vi "Delete QDFunction.vi"(8 "error in (no error)":errorcluster, 10 "QDFullName(\"\")":string, 11 "ScriptSetting in":refnum<class "ScriptSetting.lvclass">) -> (0 "error out":errorcluster, 3 "ScriptSetting out":refnum<class "ScriptSetting.lvclass">)   [LabVIEW 2015, in "ScriptSetting.lvclass"]
uses:
  ScriptSetting.lvclass
  ScriptSetting.lvclass/ScriptSetting.ctl
  QDSearchList/QDDialogList.lvclass/QDDialogList.ctl
  _Database/Implements/ScriptDatabase.lvclass/ScriptDatabase.ctl
  <vilib>/Utility/error.llb/Error Cluster From Error Code.vi
  <vilib>/ErrorRing/Error Ring.xnode
  QDSearchList/QDDialogList.lvclass
  _Database/Implements/ScriptDatabase.lvclass
  _Database/Ancestor/DatabaseAPI.lvclass
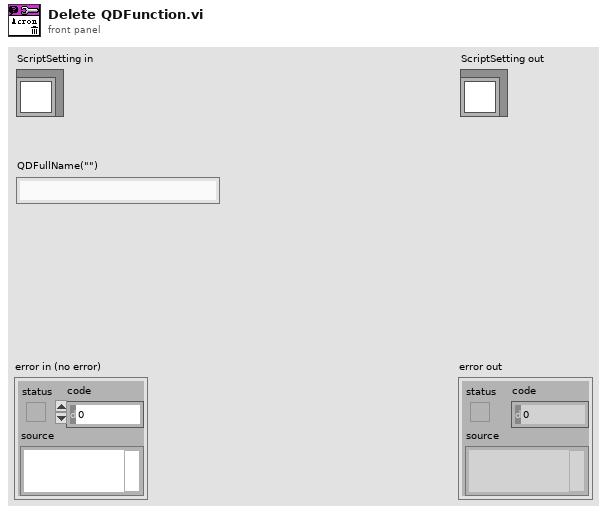
[diagram p1: front panel]
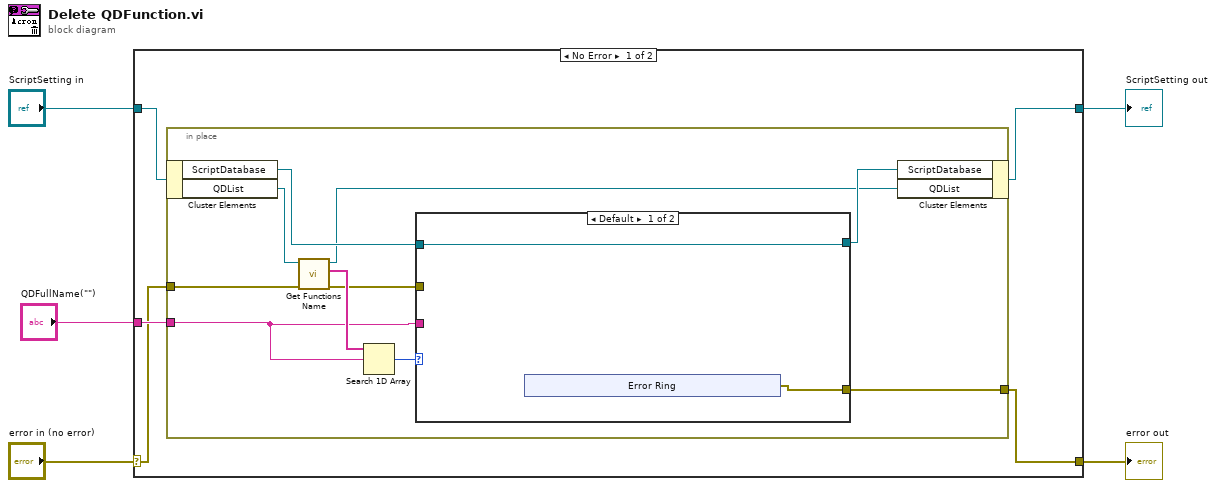
[diagram p0: block diagram]
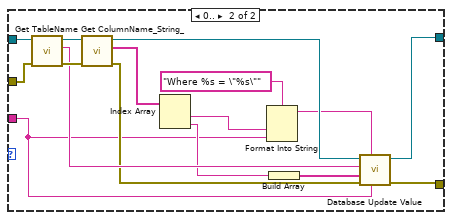
[diagram p2: hidden frame]
diagram:
  n1 = case shown="No Error" "error in (no error)" {
    selector: "error in (no error)" -> [w8 w45]
    tunnel: [w7 w45] -> w4
    tunnel: [w6 w44] -> w2
    tunnel: "ScriptSetting in" -> [w10 w44]
    tunnel: "QDFullName(\"\")" -> [w9 _]
    frame No Error {
      n2 = in-place {
        in-place-border: w9 -> [w14]
        in-place-border: w8 -> [w17]
        in-place-border: [w11] -> w7
        n3 = in-place-cluster #1(w10) -> ("ScriptDatabase"=w20:refnum<class "ScriptDatabase.lvclass">, "QDList"=w19:refnum<class "QDDialogList.lvclass">)
        n4 = call "Get Functions Name.vi"("error in (no error)"=w17, "QDDialogList in"=w19) -> ("error out"=w15:errorcluster, "Functions Name"=w18:string[], "QDDialogList out"=w12:refnum<class "QDDialogList.lvclass">)  [unwired: 7 in]
        n5 = Search 1D Array(1D array=w18, element=w14) -> (index of element=w16:i32)  [unwired: 1 in]
        n6 = case shown="Default" w16 {
          tunnel: w20 -> [w21 w42]
          tunnel: w15 -> [_ w41]
          tunnel: w14 -> [_ w29]
          tunnel: [w22 w32] -> w11
          tunnel: [w21 w28] -> w13
          frame Default {
            n7 = xnode "Error Ring"() -> ("error out"=w22:errorcluster)
          }
          frame 0.. {
            n8 = call "Get TableName.vi"("error in (no error)"=w41, "ScriptDatabase in"=w42) -> ("error out"=w39:errorcluster, "TableName"=w34:string, "ScriptDatabase out"=w40:refnum<class "ScriptDatabase.lvclass">)  [unwired: 7 in]
            n9 = call "Get ColumnName_String_.vi"("error in (no error)"=w39, "ScriptDatabase in"=w40) -> ("error out"=w33:errorcluster, "ColumnName<String>"=w38:string[], "ScriptDatabase out"=w36:refnum<class "ScriptDatabase.lvclass">)  [unwired: 7 in]
            n10 = Index Array(array=w38) -> (element #1=w37:string, element #2=w31:string)  [unwired: 2 in]
            n11 = Format Into String(format string="Where %s = \"%s\"", w37, w29) -> (resulting string=w35:string)  [unwired: 2 in, 1 out]
            n12 = Build Array(w31) -> (w30:string[])
            n13 = call "Database Update Value.vi"("data"=w29, "condition"=w35, "error in (no error)"=w33, "columns"=w30, "table"=w34, "Database in"=w36) -> ("error out"=w32:errorcluster, "Database out"=w28:refnum<class "ScriptDatabase.lvclass">)  [unwired: 4 in]
          }
        }
        n14 = in-place-cluster #1("ScriptDatabase"=w13, "QDList"=w12) -> (w6:refnum<class "ScriptSetting.lvclass">)
      }
    }
    frame Error {
    }
  }
  "error out" <- w4
  "ScriptSetting out" <- w2
